vi "ADC Data capture and Process.vi"(0 "ADC Output Read Method":T2(ring)=enum."Read .dat file", 1 "Select the Tab to project":T1(ring)=enum."ADC Sine", 2 "ADC Input":enum16{"Sine Wave", "Ramp / Triangle"}(ring), 3 "No.of samples(SNR)":i32=4096, 4 "Resolution":i32=12, 5 "active edge":i32(ring)=10280, 6 "Inputs for Dyanmic para":T9={"Fundamental Frequency"=100000.0, "Sampling Frequncy"=3999610.0, "No of Harmonics"=9, "Window"=enum."7 Term B-Harris", "Blackman (fundamental power) bins)"=1.0}, 7 "Samples per Channel":i32=4096 caption="No.of Samples(capture)", 8 "Oversampling":bool, 9 "Oversampling ratio":i32, 10 "Drop LSB":bool, 11 "Save data":T15, 12 "Waveform":i64[](array[numeric]), 13 "Path to Read":path=path "C/Users/a0230227/Desktop/save.dat", 14 "Start & Stop Bit":cluster{"Start":i32, "Stop":i32}={"Start"=40, "Stop"=4055}, 15 "length":i32=4096, 24 "path to save":T14={"Path to Save plot"=path "D/Tenor_176P/DYN_PAR_C004/DAT/D001_TEMPP30C_VDD1.2_VDDA3.3_16B_SE_ADCA__vicA_aggX_PLT_CAP_200821_1740_33.jpg", "Path to Raw Data plot"=path "D/Tenor_176P/DYN_PAR_C004/DAT/D001_TEMPP30C_VDD1.2_VDDA3.3_16B_SE_ADCA__vicA_aggX_RAW_DAT_200821_1740_33.csv"}) -> (18 "Min Max":T4, 19 "detected Throughput":dbl, 20 "output cluster":T7, 21 "Dynamic Parameters":T8, 22 "max code":ext, 23 "min code":ext, 25 "Valid Capture":bool)   [LabVIEW 2021] (continued)
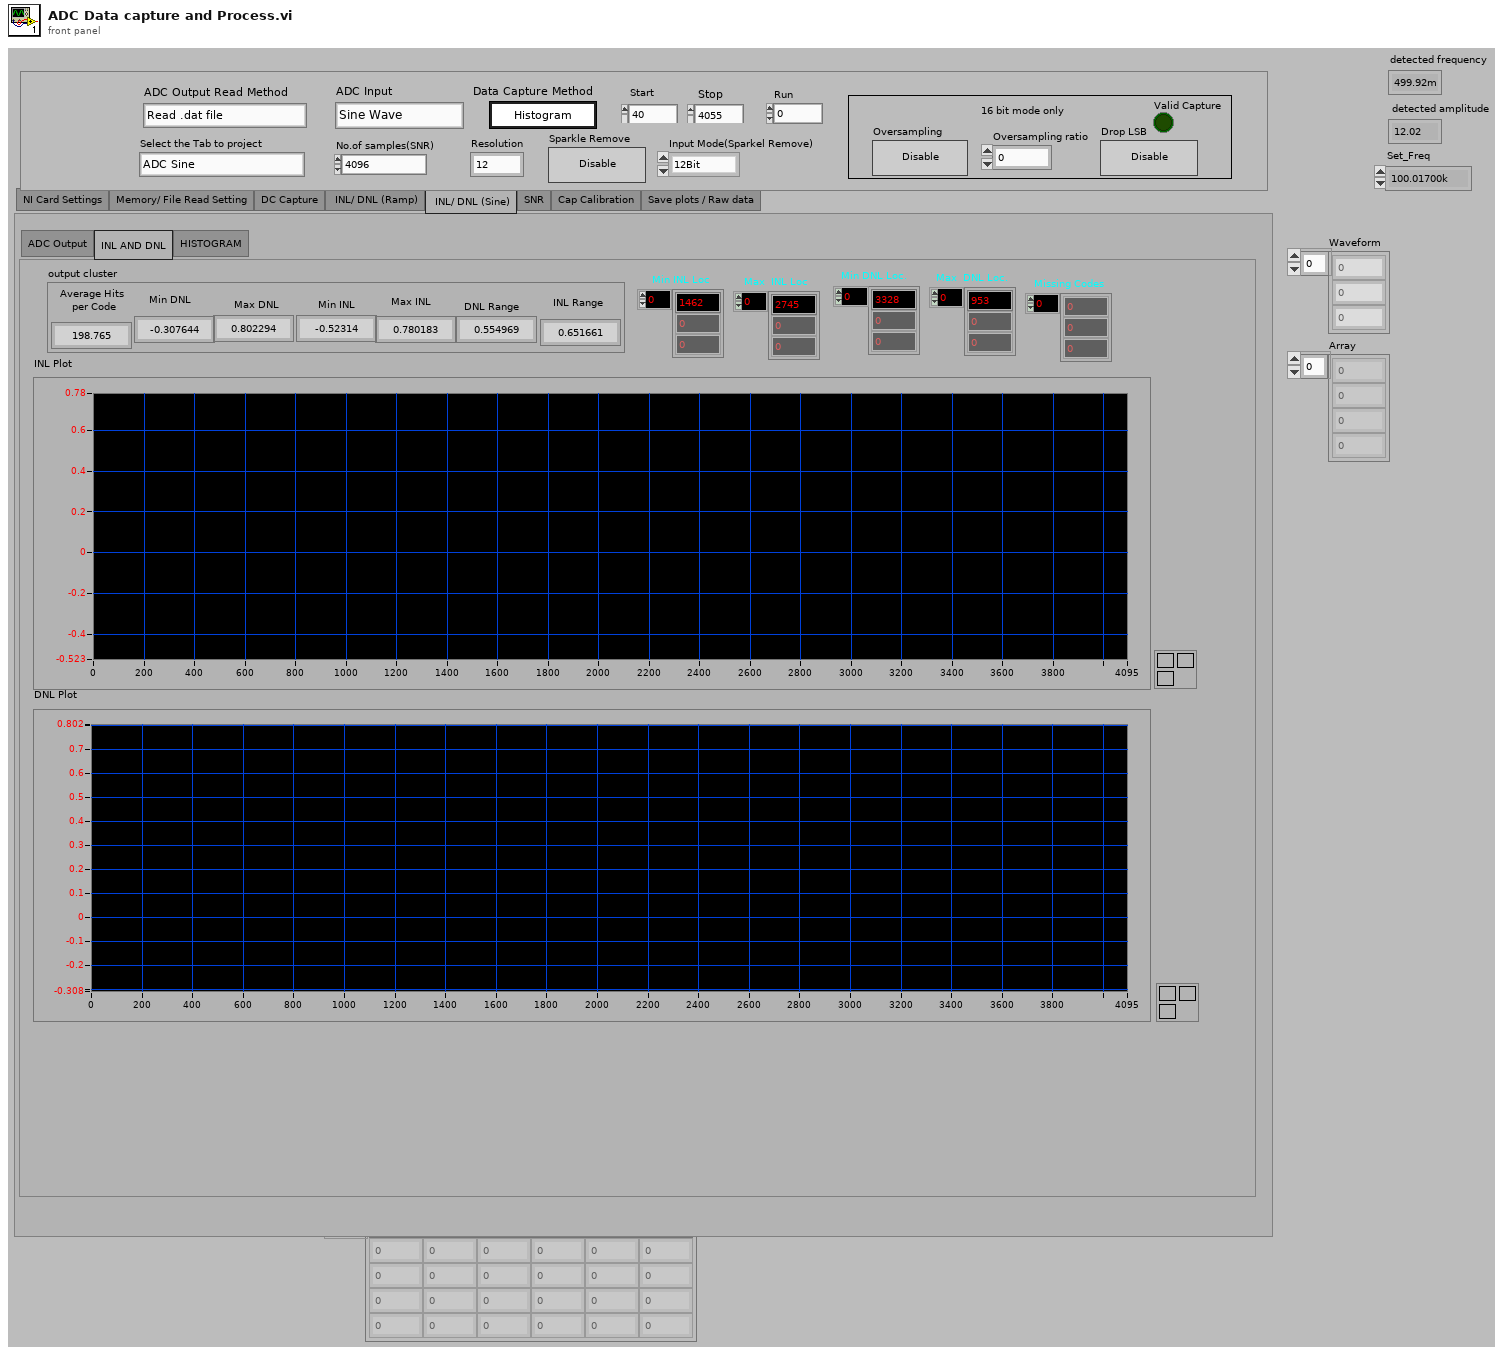
[diagram p1: front panel]
types:
  T1 = enum32{"NI Card Settings", "Memory Read Setting", "DC Capture", "ADC Ramp", "ADC Sine", "SNR", "Cap Calibration"}
  T2 = enum32{"Read from Memory", "Read .dat file", "NI Card Capture", "None"}
  T3 = enum32{"NI Card Settings", "Memory/ File Read Setting", "DC Capture", " INL/ DNL (Ramp)", " INL/ DNL (Sine)", "SNR", "Cap Calibration", "Save plots / Raw data"}
  T4 = cluster{"Min":dbl, "Max":dbl, "delta":dbl, "Average Code":dbl, "Standard Deviation":dbl}
  T5 = cluster{"Min INL":dbl, "Max INL":dbl, "Min DNL":dbl, "Max DNL":dbl, "INL Range":dbl, "DNL Range":dbl, "Avg Hits/Code":dbl}
  T6 = enum32{"ADC Output", "TRIMMED DATA", "INL AND DNL", "HISTOGRAM"}
  T7 = cluster{"Average Hits \nper Code ":dbl, "Min DNL":dbl, "Min INL":dbl, "Max INL":dbl, "Max DNL":dbl, "DNL Range":dbl, "INL Range":dbl}
  T8 = cluster{"SNR":dbl, "SNRD":dbl, "THD":dbl, "ENOB (SNRD)":dbl, "SFDR":dbl, "ENOB (SNR)":dbl, "Noise Power":dbl, "Signal power":dbl}
  T9 = cluster{"Fundamental Frequency":dbl, "Sampling Frequncy":dbl, "No of Harmonics":u8, "Window":enum16{"None ", "Hanning", "Hamming", "Blackman-Harris", "Exact Blackman", "Blackman", "Flat Top", "4 Term B-Harris ", "7 Term B-Harris"}, "Blackman (fundamental power) bins)":dbl}
  T10 = enum32{"ADC Output", "FFT Magnitude plot", " FFT plot"}
  T11 = cluster{"Ideal Power Bin":dbl, "Actual Power Bin":dbl, "Signal Strength (dB)":dbl}
  T12 = cluster{"ADC Reference(V)":dbl, "Bin Width":dbl, "PSRR/ CMRR  ":bool}
  T13 = cluster{"Fundamental Frequnecy (Calculated)":dbl, "Harmonic Frequencies":dbl[], "Harmonic Amplitudes":dbl[]}
  T14 = cluster{"Path to Save plot":path, "Path to Raw Data plot":path}
  T15 = cluster{"Save INL/DNL Plot(Ramp)":bool, "Save SNR Plot":bool, "Save INL/DNL Plot(Sine)":bool, "Save INL/DNL Raw Data(Ramp)":bool, "Save SNR Raw Data":bool, "Save INL/DNL Raw Data(Sine)":bool, "Save DC Raw data":bool, "Save  Raw Data(Sine)":bool}
  T16 = enum16{"Initialize", "Read output", "Post process", "Cap Calib", "Save data", "Exit"}
  T17 = cluster{"Average Hits \nper Code ":dbl, "Min\nDNL":dbl, dbl, dbl, "Max\nDNL":dbl, dbl, dbl}
  T18 = enum16{"None ", "Hanning", "Hamming", "Blackman-Harris", "Exact Blackman", "Blackman", "Flat Top", "4 Term B-Harris ", "7 Term B-Harris"}
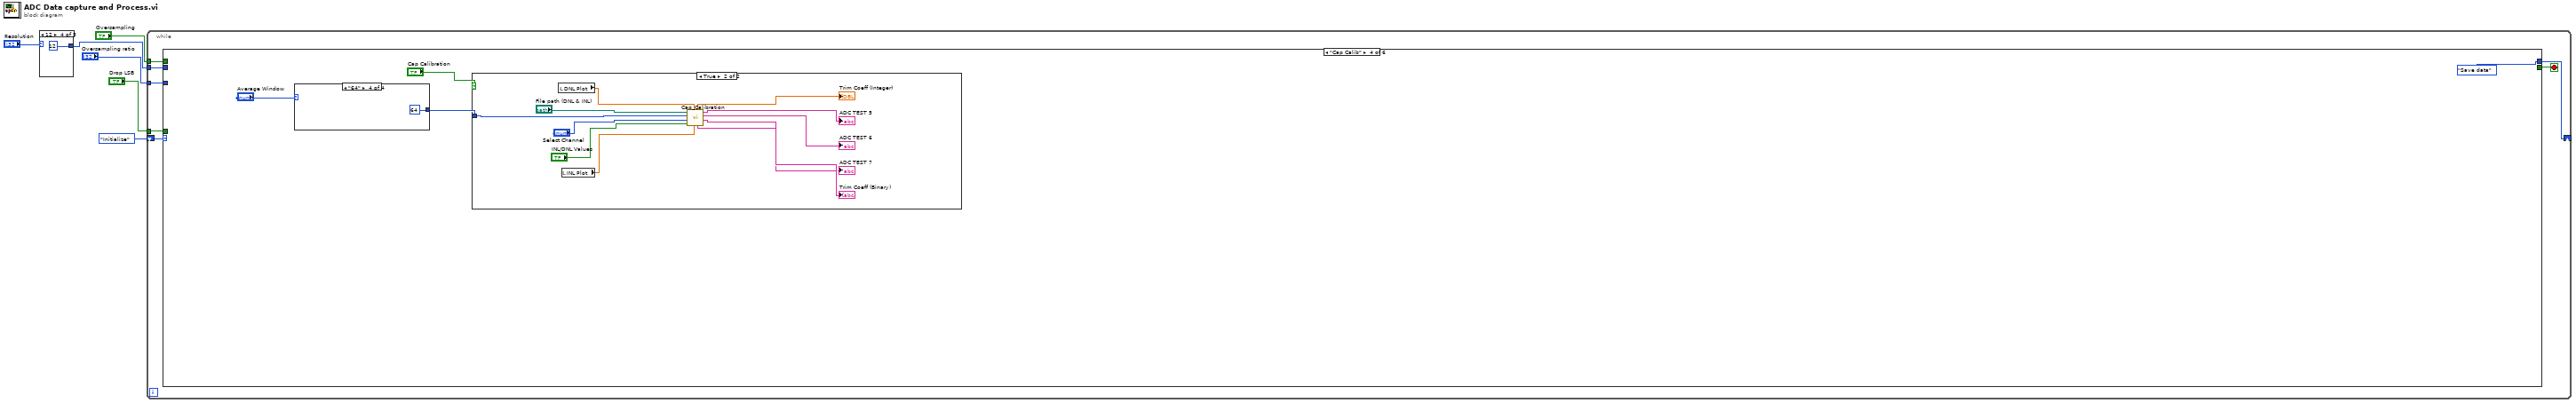
[diagram p0: block diagram]
diagram:
  n1 = case shown="12" "Resolution" {
    tunnel: [18 16 14 12 10] -> w5
    frame 18 {
    }
    frame 16 {
    }
    frame 14, Default {
    }
    frame 12 {
    }
    frame 10 {
    }
  }
  n2 = while {
    shift-right: [w17] -> _
    shift-left: T16."Initialize" -> [w18]
    tunnel: w5 -> [w15]
    tunnel: "Oversampling" -> [w14]
    tunnel: "Drop LSB" -> [w13]
    tunnel: "Oversampling ratio" -> [w12]
    stop <- w16 stop-if-true
    n3 = case shown="\"Cap Calib\"" w18 {
      tunnel: [T16."Read output" w41 w114 T16."Save data" T16."Exit" _] -> w17
      tunnel: [_ _ _ _ _ TRUE] -> w16
      tunnel: w15 -> [_ _ w121 _ _ _]
      tunnel: w14 -> [_ _ w111 _ _ _]
      tunnel: w13 -> [_ _ w113 _ _ _]
      tunnel: w12 -> [_ _ w112 _ _ _]
      frame "Initialize", Default {
        n4 = local read "No.of samples(SNR)"() -> (w19:i32)
        n5 = local write "Samples per Channel"(w19) -> ()
      }
      frame "Read output" {
        w26 = waveform(i64) {"t0"=timestamp(0 s since 1904-01-01), "dt"=1.0, "Y"=[]}  # waveform
        n6 = case shown="\"NI Card Capture\", Default" "ADC Output Read Method" {
          tunnel: [w51 _ w70 "Waveform"] -> w27
          tunnel: [T16."Post process" _ T16."Post process" T16."Post process"] -> w41
          frame "Read .dat file" {
            w50 = 0  # index
            w56 = 8192 ("index")
            w61 = 1 ("index")
            n7 = call-poly <vilib>:"Read From Spreadsheet File.vi"("delimiter (\\t)"="Delimiter (\\t)", "file path (dialog if empty)"="Path to Read") -> ("all rows"=w63:i64[][])  [unwired: 5 in, 4 out]
            n8 = Index Array(array=w63, index (col)=0 ("disabled index (col)")) -> (element=w54:i64[])  [unwired: 1 in]
            n9 = Split 1D Array(array=w54, index=w61) -> (second subarray=w52:i64[])  [unwired: 1 out]
            n10 = Multiply(x=w56, y=1) -> (x*y=w59:i32)
            n11 = Multiply(x=2 ("y"), y=w56) -> (x*y=w57:i32)
            n12 = Multiply(x=w56, y=3) -> ()  [unwired: 1 out]
            n13 = Array Subset(array=w52, index=w61, length=w56) -> ()  [unwired: 1 out]
            n14 = Array Subset(array=w52, index=w59, length=w56) -> ()  [unwired: 1 out]
            n15 = Array Subset(array=w52, index=w57, length=w56) -> ()  [unwired: 1 out]
            n16 = Array Subset(array=w52, index=w50, length="length") -> (w51:i64[])
          }
          frame "None" {
          }
          frame "NI Card Capture", Default {
            n17 = case shown="\"Sine Wave\", Default" "ADC Input" {
              tunnel: "Port" -> [w87 w97]
              tunnel: "Source" -> [w86 w96]
              tunnel: "Rate" -> [w85 w95]
              tunnel: "Timeout" -> [w84 w94]
              tunnel: [_ w92] -> w69
              tunnel: [w80 w93] -> w70
              tunnel: "No.of samples(SNR)" -> [w83 w91]
              tunnel: "Samples per Channel" -> [w81 w90]
              tunnel: "Sparkle Remove" -> [w79 _]
              tunnel: "active edge" -> [w78 w88]
              frame "Sine Wave", Default {
                n18 = call "DATA_CAPTURE_SNR.vi"("Port"=w87, "Source"=w86, "No. of samples to process"=w83, "Samples per Channel"=w81, "Rate"=w85, "active edge"=w78, "timeout"=w84, "Histogram Capture Method SNR"=w79, "NI card Cont/Single Capture"=FALSE ("Histogram Capture Method SNR")) -> ("Waveform"=w80:u32[])  [unwired: 5 in, 5 out]
              }
              frame "Ramp / Triangle" {
                n19 = disable-structure shown="Disabled" {
                  disable-tunnel: w97 -> [w108 _]
                  disable-tunnel: w96 -> [w107 _]
                  disable-tunnel: w95 -> [w106 _]
                  disable-tunnel: w94 -> [w105 _]
                  disable-tunnel: [w104 _] -> w93
                  disable-tunnel: [w103 _] -> w92
                  disable-tunnel: w91 -> [w102 _]
                  disable-tunnel: w90 -> [w100 _]
                  disable-tunnel: FALSE ("Histogram Capture Method SNR") -> [w99 _]
                  disable-tunnel: w88 -> [w98 _]
                  frame Disabled {
                    n20 = call "DATA_CAPTURE_SNR.vi"("Port"=w108, "Source"=w107, "No. of samples to process"=w102, "Samples per Channel"=w100, "Rate"=w106, "active edge"=w98, "timeout"=w105, "Histogram Capture Method SNR"=w99, "NI card Cont/Single Capture"=FALSE ("Histogram Capture Method SNR")) -> ("Waveform"=w104:u32[], "Trimmed Wave"=w103:u32[])  [unwired: 5 in, 4 out]
                  }
                  frame Enabled {
                  }
                }
              }
            }
            "Trimmed Wave" <- w69
          }
          frame "Read from Memory" {
          }
        }
        "Ramp Waveform" <- w27
        "Sine Waveform" <- w27
        "Read Data from Device" <- w27
        "Captured Data" <- w27
        "DC capture" <- w27
        n21 = Bundle By Name(cluster=w26, "Y"=w27) -> (w25:waveform(i64))
        n22 = Array Size(array=w27) -> (size(s)=w37:i32)
        n23 = Array Max & Min(array=w27) -> (max value=→"max code":i64, min value=→"min code":i64)  [unwired: 2 out]
        n24 = Decrement(x=w37) -> (x-1=w36:i32)
        n25 = call-poly <vilib>:"Extract Single Tone Information.vi"("time signal in"=w25) -> ("detected amplitude"=→"detected amplitude":dbl, "detected frequency"=w22:dbl)  [unwired: 5 in, 4 out]
        "detected frequency" <- w22
        n26 = for {
          N: w36 -> [_]
          tunnel: w27 -> [w48]
          tunnel: [w42] -> w34 mode=indexing
          i -> [w46]
          n27 = Increment(x=w46) -> (x+1=w47:i32)
          n28 = Index Array(array=w48, index=w46) -> (element=w44:i64)
          n29 = Index Array(array=w48, index=w47) -> (element=w45:i64)
          n30 = Subtract(x=w45, y=w44) -> (x-y=w43:i64)
          n31 = Absolute Value(x=w43) -> (abs(x)=w42:i64)
        }
        n32 = Divide(x="Set_Freq", y=w22) -> (x/y=→"detected Throughput":dbl)
        n33 = Add Array Elements(numeric array=w34) -> (sum=w32:i64)
        n34 = Array Max & Min(array=w34) -> (max value=w29:i64)  [unwired: 3 out]
        n35 = Array Size(array=w34) -> (size(s)=w31:i32)
        n36 = Divide(x=w32, y=w31) -> (x/y=w33:dbl)
        n37 = Multiply(x=2.0, y=w33) -> (x*y=w28:dbl)
        n38 = Less?(x=w29, y=w28) -> (x < y?=→"Valid Capture":bool)
      }
      frame "Post process" {
        n39 = local read "Select the Tab to project"() -> (w127:T1)
        n40 = local read "Read Data from Device"() -> (w118:dbl[])
        n41 = local read "No.of samples(SNR)"() -> (w120:i32)
        n42 = Equal?(x=w127, y=T1."Cap Calibration" ("Select the Tab to project")) -> (x = y?=w128:bool)
        n43 = Unbundle By Name("Start & Stop Bit") -> ("Start"=w123:i32, "Stop"=w122:i32)
        n44 = Select(t=T1."ADC Sine" ("Select the Tab to project"), s=w128, f=w127) -> (s? t:f=w126:T1)
        n45 = case shown="\"SNR\"" w126 {
          tunnel: w118 -> [w133 w249 w321 w386]
          tunnel: "Data Capture Method" -> [w130 w247 w354 _]
          tunnel: w123 -> [_ w246 w353 _]
          tunnel: w122 -> [_ w245 w352 _]
          tunnel: w121 -> [_ w248 w351 w385]
          tunnel: w120 -> [_ _ _ w387]
          tunnel: [_ w244 w339 _] -> w119
          tunnel: [T16."Save data" T16."Save data" T16."Cap Calib" T16."Save data"] -> w114
          tunnel: w111 -> [_ _ w318 w383]
          tunnel: w113 -> [_ _ w317 w382]
          tunnel: w112 -> [_ _ w319 w381]
          frame "DC Capture", Default {
            n46 = property on="Raw Data CH2" class="Arr (strict)"("Visible"="CH Swtich (To see other CH O/P)") -> ()  [unwired: 2 in, 2 out]
            n47 = property on="Standard Deviation (CH2)" class="DigNum (strict)"("Visible"="CH Swtich (To see other CH O/P)") -> ()  [unwired: 2 in, 2 out]
            n48 = property on="Raw Data CH1" class="Arr (strict)"("Visible"="CH Swtich (To see other CH O/P)") -> ()  [unwired: 2 in, 2 out]
            n49 = property on="Average Code (CH2)" class="DigNum (strict)"("Visible"="CH Swtich (To see other CH O/P)") -> ()  [unwired: 2 in, 2 out]
            n50 = case shown="False" w130 {
              tunnel: w133 -> [w136 w204]
              tunnel: "CH Swtich (To see other CH O/P)" -> [w135 _]
              tunnel: [w134 w190] -> w129
              frame False {
                n51 = case shown="True" w135 {
                  tunnel: w136 -> [w141 w178]
                  tunnel: [w137 w170] -> w134
                  frame True {
                    w147 = 10 ("index")
                    w160 = 10 ("index")
                    n52 = Decimate 1D Array(w141) -> (w157:dbl[], w148:dbl[])
                    "Raw Data CH2" <- w157
                    "Raw Data CH1" <- w148
                    n53 = Split 1D Array(array=w157, index=w160) -> (second subarray=w159:dbl[])  [unwired: 1 out]
                    n54 = Split 1D Array(array=w148, index=w147) -> (second subarray=w156:dbl[])  [unwired: 1 out]
                    n55 = Array Size(array=w159) -> (size(s)=w161:i32)
                    n56 = Array Size(array=w156) -> (size(s)=w155:i32)
                    n57 = Subtract(x=w161, y=w160) -> (x-y=w164:i32)
                    n58 = Subtract(x=w155, y=w147) -> (x-y=w145:i32)
                    n59 = Split 1D Array(array=w159, index=w164) -> (first subarray=w163:dbl[])  [unwired: 1 out]
                    n60 = Split 1D Array(array=w156, index=w145) -> (first subarray=w153:dbl[])  [unwired: 1 out]
                    n61 = Array Size(array=w163) -> (size(s)=w162:i32)
                    n62 = Array Size(array=w153) -> (size(s)=w154:i32)
                    n63 = To Double Precision Float(number=w163) -> (double precision float=w165:dbl[])
                    n64 = To Double Precision Float(number=w153) -> (double precision float=w144:dbl[])
                    n65 = Add Array Elements(numeric array=w165) -> (sum=w169:dbl)
                    n66 = Add Array Elements(numeric array=w144) -> (sum=w149:dbl)
                    n67 = Divide(x=w169, y=w162) -> (x/y=w142:dbl)
                    "Average Code (CH2)" <- w142
                    n68 = Divide(x=w149, y=w154) -> (x/y=w139:dbl)
                    n69 = Subtract(x=w165, y=w142) -> (x-y=w168:dbl[])
                    n70 = Subtract(x=w144, y=w139) -> (x-y=w150:dbl[])
                    n71 = Square(x=w168) -> (x^2=w167:dbl[])
                    n72 = Square(x=w150) -> (x^2=w151:dbl[])
                    n73 = Add Array Elements(numeric array=w167) -> (sum=w166:dbl)
                    n74 = Add Array Elements(numeric array=w151) -> (sum=w152:dbl)
                    n75 = Divide(x=w166, y=w162) -> (x/y=w158:dbl)
                    n76 = Divide(x=w152, y=w154) -> (x/y=w146:dbl)
                    n77 = Square Root(x=w158) -> (sqrt(x)=→"Standard Deviation (CH2)":dbl)
                    n78 = Square Root(x=w146) -> (sqrt(x)=w138:dbl)
                    n79 = local read "Min Max"() -> (w140:T4)
                    n80 = Bundle By Name(cluster=w140, "Average Code"=w139, "Standard Deviation"=w138) -> (w137:T4)
                  }
                  frame False {
                    w182 = 10 ("index")
                    n81 = Split 1D Array(array=w178, index=w182) -> (second subarray=w189:dbl[])  [unwired: 1 out]
                    n82 = Array Size(array=w189) -> (size(s)=w188:i32)
                    n83 = Subtract(x=w188, y=w182) -> (x-y=w180:i32)
                    n84 = Split 1D Array(array=w189, index=w180) -> (first subarray=w177:dbl[])  [unwired: 1 out]
                    n85 = Array Size(array=w177) -> (size(s)=w187:i32)
                    n86 = To Double Precision Float(number=w177) -> (double precision float=w179:dbl[])
                    n87 = Add Array Elements(numeric array=w179) -> (sum=w183:dbl)
                    n88 = Divide(x=w183, y=w187) -> (x/y=w172:dbl)
                    n89 = Subtract(x=w179, y=w172) -> (x-y=w184:dbl[])
                    n90 = Square(x=w184) -> (x^2=w185:dbl[])
                    n91 = Add Array Elements(numeric array=w185) -> (sum=w186:dbl)
                    n92 = Divide(x=w186, y=w187) -> (x/y=w181:dbl)
                    n93 = Array Max & Min(array=w177) -> (max value=w174:dbl, min value=w173:dbl)  [unwired: 2 out]
                    n94 = local read "Min Max"() -> (w176:T4)
                    n95 = Subtract(x=w174, y=w173) -> (x-y=w175:dbl)
                    n96 = Square Root(x=w181) -> (sqrt(x)=w171:dbl)
                    n97 = Bundle By Name(cluster=w176, "Standard Deviation"=w171, "Average Code"=w172, "Max"=w174, "Min"=w173, "delta"=w175) -> (w170:T4)
                  }
                }
              }
              frame True {
                n98 = for {
                  tunnel: w204 -> [w237] mode=indexing
                  shift-right: [w241] -> w213
                  shift-left: 0.0 ("x*y") -> [w242]
                  tunnel: w204 -> [w240]
                  tunnel: [w239] -> w212
                  shift-right: [w228] -> _
                  shift-left: TRUE ("x != 0?") -> [w235]
                  shift-right: [w231] -> w195
                  shift-left: i32[] [] -> [w232]
                  i -> [w234]
                  n99 = Add Array Elements(numeric array=w240) -> (sum=w239:dbl)
                  n100 = Not Equal To 0?(x=w237) -> (x != 0?=w236:bool)
                  n101 = Multiply(x=w237, y=w234) -> (x*y=w238:dbl)
                  n102 = Build Array (concatenate)(w232, w234) -> (w233:i32[])
                  n103 = And(x=w235, y=w236) -> (x .and. y?=w230:bool)
                  n104 = Add(x=w242, y=w238) -> (x+y=w241:dbl)
                  n105 = Select(t=w233, s=w230, f=w232) -> (s? t:f=w231:i32[])
                  n106 = Select(t=FALSE ("x != 0?"), s=w230, f=TRUE ("x != 0?")) -> (s? t:f=w228:bool)
                }
                n107 = Divide(x=w213, y=w212) -> (x/y=w191:dbl)
                n108 = Array Size(array=w195) -> (size(s)=w193:i32)
                n109 = Index Array(array=w195, index=0) -> (element=w196:i32)
                n110 = Split 1D Array(array=w204, index=w196) -> (second subarray=w199:dbl[])  [unwired: 1 out]
                n111 = Subtract(x=w193, y=15 ("x")) -> (x-y=w192:i32)
                n112 = Array Max & Min(array=w199) -> (max index (indices)=w207:i32)  [unwired: 3 out]
                n113 = Greater?(x=w207, y=w192) -> (0:w208:bool)
                n114 = case shown="True" w208 {
                  tunnel: w207 -> [w216 w223]
                  tunnel: [w215 w223] -> w203
                  tunnel: 10 ("y") -> [w220 w222]
                  tunnel: w199 -> [w219 w226]
                  tunnel: [w216 w225] -> w202
                  tunnel: [_ w221] -> w197
                  frame True {
                    n115 = Subtract(x=w216, y=w220) -> (x-y=w217:i32)
                    n116 = Split 1D Array(array=w219, index=w217) -> (first subarray=w218:dbl[])  [unwired: 1 out]
                    n117 = Array Max & Min(array=w218) -> (max index (indices)=w215:i32)  [unwired: 3 out]
                  }
                  frame False {
                    n118 = Add(x=w223, y=w222) -> (x+y=w221:i32)
                    n119 = Split 1D Array(array=w226, index=w221) -> (second subarray=w224:dbl[])  [unwired: 1 out]
                    n120 = Array Max & Min(array=w224) -> (max index (indices)=w225:i32)  [unwired: 3 out]
                  }
                }
                n121 = Add(x=w196, y=w203) -> (x+y=w200:i32)
                n122 = Compound Arithmetic op=ADD(w196, w202, w197) -> (w201:i32)
                n123 = Subtract(x=w201, y=w200) -> (x-y=w206:i32)
                n124 = local read "Min Max"() -> (w211:T4)
                n125 = Bundle By Name(cluster=w211, "Average Code"=w191, "Min"=w200, "Max"=w201, "delta"=w206) -> (w190:T4)
              }
            }
            "Min Max" <- w129
          }
          frame "ADC Ramp" {
            n126 = stacked-sequence {
              seq-local: [w251 _ _] -> [_ w275 _]
              seq-local: [_ w271 _] -> [_ _ w301]
              seq-local: [_ w270 _] -> [_ _ w300]
              seq-local: [_ w269 _] -> [_ _ w289]
              seq-local: [w252 _ _] -> [_ w268 _]
              tunnel: w249 -> [w254 _ _]
              tunnel: w248 -> [w256 _ _]
              tunnel: w247 -> [w255 _ _]
              tunnel: w246 -> [_ w274 _]
              tunnel: w245 -> [_ w273 _]
              tunnel: [w251 _ _] -> w244
              frame #0 {
                n127 = local read "Trimmed Wave"() -> (w250:u32[])
                n128 = Scale By Power Of 2(n=w256, x=ext 1.0) -> (x*2^n=w252:ext)
                n129 = Initialize Array(0 ("element"), w252) -> (w260:i32[])
                n130 = for {
                  shift-right: [w263] -> w253
                  shift-left: w260 -> [w264]
                  tunnel: 0.0 -> [w262]
                  tunnel: w250 -> [w261] mode=indexing
                  n131 = Subtract(x=w261, y=w262) -> (x-y=w265:dbl)
                  n132 = in-place {
                    n133 = in-place-array #1(w264, w265) -> (w267:i32)
                    n134 = Increment(x=w267) -> (x+1=w266:i32)
                    n135 = in-place-array #1(w266) -> (w263:i32[])  [unwired: 1 out]
                  }
                }
                n136 = Select(t=w254, s=w255, f=w253) -> (s? t:f=w251:dbl[])
                "Histogram waveform" <- w251
              }
              frame #1 {
                n137 = Subtract(x=w273, y=w274) -> (x-y=w276:i32)
                n138 = Split 1D Array(array=w275, index=w274) -> (second subarray=w283:dbl[])  [unwired: 1 out]
                n139 = Split 1D Array(array=w283, index=w276) -> (first subarray=w277:dbl[])  [unwired: 1 out]
                n140 = Add Array Elements(numeric array=w277) -> (sum=w280:dbl)
                n141 = Array Size(array=w277) -> (size(s)=w279:i32)
                n142 = Divide(x=w280, y=w279) -> (x/y=w269:dbl)
                n143 = Initialize Array(w269, w268) -> (w278:dbl[])
                n144 = Replace Array Subset(array=w278, new element=w277, index=w274) -> (w282:dbl[])
                n145 = Divide(x=w282, y=w269) -> (x/y=w281:dbl[])
                n146 = Decrement(x=w281) -> (x-1=w271:dbl[])
                "DNL_Ramp" <- w271
                n147 = for {
                  shift-right: [w285] -> _
                  shift-left: 0.0 ("x") -> [w286]
                  tunnel: [w285] -> w270 mode=indexing
                  tunnel: w271 -> [w284] mode=indexing
                  n148 = Add(x=w286, y=w284) -> (x+y=w285:dbl)
                }
                "INL_Ramp" <- w270
              }
              frame #2 {
                n149 = Array Max & Min(array=w301) -> (max value=w292:dbl, min value=w293:dbl)  [unwired: 2 out]
                n150 = Array Max & Min(array=w300) -> (max value=w294:dbl, min value=w295:dbl)  [unwired: 2 out]
                n151 = Subtract(x=w292, y=w293) -> (x-y=w297:dbl)
                n152 = Subtract(x=w294, y=w295) -> (x-y=w298:dbl)
                n153 = local read "Static Parameters (Ramp)"() -> (w288:T5)
                n154 = Divide(x=w297, y=2.0) -> (x/y=w290:dbl)
                n155 = Divide(x=w298, y=2.0) -> (x/y=w291:dbl)
                n156 = disable-structure shown="Enabled" {
                  disable-tunnel: w295 -> [w316 _]
                  disable-tunnel: w294 -> [w315 _]
                  disable-tunnel: w293 -> [w314 _]
                  disable-tunnel: w292 -> [w313 _]
                  disable-tunnel: w291 -> [w304 _]
                  disable-tunnel: w290 -> [w303 _]
                  disable-tunnel: w289 -> [w302 _]
                  frame Disabled {
                    n157 = Increment(x="Run") -> (x+1=w305:dbl)
                    n158 = local write "Run"(w305) -> ()
                    n159 = Build Array(w305, w316, w315, w314, w313, w304, w303, w302) -> (w312:dbl[])
                    n160 = call-poly <vilib>:"Write To Spreadsheet File.vi"("delimiter (\\t)"="," ("delimiter (\\t)"), "transpose? (no:F)"=FALSE, "format (%.3f)"="%.4f", "append to file? (new file:F)"=TRUE, "1D data"=w312, "file path (dialog if empty)"=path "D:/FALCON/ADC/Raw_Data/runtorun.csv") -> ()  [unwired: 2 in, 1 out]
                  }
                  frame Enabled {
                  }
                }
                n161 = Bundle By Name(cluster=w288, "Max INL"=w294, "Min INL"=w295, "Max DNL"=w292, "Min DNL"=w293, "INL Range"=w291, "DNL Range"=w290, "Avg Hits/Code"=w289) -> (→"Static Parameters (Ramp)":T5)
              }
            }
          }
          frame "ADC Sine" {
            n162 = case shown="True" w318 {
              tunnel: w321 -> [w356 w364]
              tunnel: [w357 w362] -> w320
              tunnel: w319 -> [_ w363]
              tunnel: w317 -> [w355 _]
              frame False {
                n163 = case shown="True" w355 {
                  tunnel: w356 -> [w358 w360]
                  tunnel: [w358 w359] -> w357
                  frame False {
                  }
                  frame True {
                    n164 = Divide(x=w360, y=2.0) -> (x/y=w359:dbl[])
                  }
                }
              }
              frame True {
                n165 = Array Size(array=w364) -> (size(s)=w366:i32)
                n166 = Divide(x=w366, y=w363) -> (x/y=w365:dbl)
                n167 = for {
                  N: w365 -> [_]
                  tunnel: w364 -> [w373]
                  tunnel: w363 -> [w368]
                  tunnel: [w367] -> w362 mode=indexing
                  i -> [w372]
                  n168 = Multiply(x=w368, y=w372) -> (x*y=w371:i32)
                  n169 = Array Subset(array=w373, index=w371, length=w368) -> (w370:dbl[])
                  n170 = Add Array Elements(numeric array=w370) -> (sum=w369:dbl)
                  n171 = Divide(x=w369, y=w368) -> (x/y=w367:dbl)
                }
              }
            }
            n172 = call "Sinewave_Linearity_trial_F027.vi"("Array"=w320, "Histogram Capture Method"=w354, "L code"=w353, "UCode"=w352, "Resolution"=w351, "Histogram: h(x)"=w320) -> ("Average Hits \nper Code"=w329:dbl, "Max\nDNL"=w325:dbl, "Min\nDNL"=w328:dbl, "Missing Codes"=→"Missing Codes":i32[], "Max  DNL Loc."=→"Max  DNL Loc.":i32[], "Min DNL Loc."=→"Min DNL Loc.":i32[], "Max  INL Loc"=→"Max  INL Loc":i32[], "Min INL Loc"=→"Min INL Loc":i32[], "Histogram Plot"=w341:dbl[][], "DNL Plot"=w337:dbl[], "INL Plot"=w330:dbl[])  [unwired: 1 in, 2 out]
            "Histogram Plot" <- w341
            "DNL Plot" <- w337
            "INL Plot" <- w330
            n173 = for {
              tunnel: w337 -> [w380] mode=indexing
              tunnel: [w376] -> w336 mode=indexing
              shift-right: [w375] -> _
              shift-left: 16384 ("f") -> [w374]
              i -> [w377]
              n174 = Increment(x=w374) -> (x+1=w375:i32)
              n175 = Greater?(x=w380, y=0.9) -> (0:w378:bool)
              n176 = Select(t=w377, s=w378, f=w374) -> (s? t:f=w376:i32)
            }
            n177 = Subtract(x=w325, y=w328) -> (x-y=w348:dbl)
            n178 = Array Max & Min(array=w330) -> (max value=w326:dbl, min value=w327:dbl)  [unwired: 2 out]
            n179 = Index Array(array=w341, index (col)=1 ("disabled index (col)")) -> (element=w339:dbl[])  [unwired: 1 in]
            n180 = Subtract(x=w326, y=w327) -> (x-y=w350:dbl)
            n181 = Divide(x=w348, y=2.0) -> (x/y=w324:dbl)
            n182 = Divide(x=w350, y=2.0) -> (x/y=w323:dbl)
            n183 = Bundle("Average Hits \nper Code"=w329, "Min\nDNL"=w328, w327, w326, "Max\nDNL"=w325, w324, w323) -> (→"output cluster":T17)  [unwired: 1 in]
            n184 = Sort 1D Array(array=w336) -> (sorted array=w332:i32[])
            n185 = Search 1D Array(1D array=w332, element=16384) -> (index of element=w333:i32)  [unwired: 1 in]
            n186 = Array Subset(array=w332, length=w333) -> (→"Array":i32[])  [unwired: 1 in]
          }
          frame "SNR" {
            n187 = stacked-sequence {
              seq-local: [w408 _ _] -> [_ w469 _]
              seq-local: [w407 _ _] -> [_ _ w494]
              seq-local: [w401 _ _] -> [_ _ w497]
              seq-local: [w400 _ _] -> [_ _ w493]
              seq-local: [w399 _ _] -> [_ _ w492]
              tunnel: w387 -> [w420 _ w495]
              tunnel: w386 -> [w402 _ _]
              tunnel: w385 -> [w404 _ _]
              tunnel: w383 -> [w391 _ _]
              tunnel: w382 -> [w390 _ _]
              tunnel: w381 -> [w389 _ _]
              frame #0 {
                n188 = Unbundle By Name("PSRR/CMRR Input") -> ("ADC Reference(V)"=w403:dbl, "PSRR/ CMRR"=w399:bool)
                n189 = case shown="True" w399 {
                  tunnel: 1.0 ("x") -> [_ w455]
                  tunnel: w404 -> [_ w454]
                  tunnel: w403 -> [_ w452]
                  tunnel: w402 -> [w448 w450]
                  tunnel: [w448 w449] -> w393
                  frame False {
                  }
                  frame True {
                    n190 = Scale By Power Of 2(n=w454, x=w455) -> (x*2^n=w453:dbl)
                    n191 = Divide(x=w452, y=w453) -> (x/y=w451:dbl)
                    n192 = Multiply(x=w450, y=w451) -> (x*y=w449:dbl[])
                  }
                }
                n193 = case shown="True" w391 {
                  tunnel: w393 -> [w430 w438]
                  tunnel: [w431 w436] -> w392
                  tunnel: w389 -> [_ w437]
                  tunnel: w390 -> [w429 _]
                  frame False {
                    n194 = case shown="True" w429 {
                      tunnel: w430 -> [w432 w434]
                      tunnel: [w432 w433] -> w431
                      frame False {
                      }
                      frame True {
                        n195 = Divide(x=w434, y=2.0) -> (x/y=w433:dbl[])
                      }
                    }
                  }
                  frame True {
                    n196 = Array Size(array=w438) -> (size(s)=w440:i32)
                    n197 = Divide(x=w440, y=w437) -> (x/y=w439:dbl)
                    n198 = for {
                      N: w439 -> [_]
                      tunnel: w438 -> [w447]
                      tunnel: w437 -> [w442]
                      tunnel: [w441] -> w436 mode=indexing
                      i -> [w446]
                      n199 = Multiply(x=w442, y=w446) -> (x*y=w445:i32)
                      n200 = Array Subset(array=w447, index=w445, length=w442) -> (w444:dbl[])
                      n201 = Add Array Elements(numeric array=w444) -> (sum=w443:dbl)
                      n202 = Divide(x=w443, y=w442) -> (x/y=w441:dbl)
                    }
                  }
                }
                n203 = Unbundle By Name("Inputs for Dyanmic para") -> ("Window"=w418:T18, "Sampling Frequncy"=w407:dbl, "Fundamental Frequency"=w401:dbl, "No of Harmonics"=w408:u8, "Blackman (fundamental power) bins)"=w417:dbl)
                n204 = Reciprocal(x=w407) -> (1/x=w422:dbl)
                n205 = call-poly <vilib>:"Scaled Time Domain Window.vi"("window"=w418, "X"=w392) -> ("Windowed X"=w426:dbl[])  [unwired: 7 in, 2 out]
                n206 = local read "Dynamic Parameters"() -> (w416:T8)
                n207 = call <vilib>:"Auto Power Spectrum.vi"("dt"=w422, "Signal (V)"=w426) -> ("Power Spectrum (V^2 rms)"=w421:dbl[])  [unwired: 1 out]
                n208 = Logarithm Base 10(1:w421) -> (0:w428:dbl[])
                n209 = call "Calculate_SNR_THD.vi"("Auto Power Spectrum"=w421, "frame size"=w420, "# harmonics"=w408, "window"=w418, "sampling rate"=w407, "fundamental frequency"=w401, "Blackman\n (fundamental power bins)"=w417) -> ("% THD"=w415:dbl, "ENOB(SNRD)"=w410:dbl, "% THD + Noise"=w388:dbl, "ENOB(SNR)"=w411:dbl, "Noise Power"=w414:dbl, "Fundamental frequency Calculated"=w396:dbl, "SNR"=w413:dbl, "Signal power"=w412:dbl, "Harmonic Amplitudes"=w423:dbl[], "Harmonic Frequencies"=w398:dbl[])  [unwired: 3 in]
                n210 = Bundle By Name(cluster=w416, "THD"=w415, "SNRD"=w388, "Noise Power"=w414, "SNR"=w413, "Signal power"=w412, "ENOB (SNR)"=w411, "ENOB (SNRD)"=w410) -> (→"Dynamic Parameters":T8)
                n211 = Logarithm Base 10(1:w423) -> (0:w425:dbl[])
                n212 = Multiply(x=10.0, y=w428) -> (x*y=w400:dbl[])
                "FFT Magnitude Plot (dB)" <- w400
                n213 = local read "Harmonic Details"() -> (w394:T13)
                n214 = Multiply(x=20, y=w425) -> (x*y=w397:dbl[])
                n215 = Bundle By Name(cluster=w394, "Fundamental Frequnecy (Calculated)"=w396, "Harmonic Frequencies"=w398, "Harmonic Amplitudes"=w397) -> (→"Harmonic Details":T13)
              }
              frame #1 {
                n216 = local read "Harmonic Details"() -> (w457:T13)
                n217 = Unbundle By Name(w457) -> ("Harmonic Amplitudes"=w456:dbl[])
                n218 = Decrement(x=w469) -> (x-1=w475:u8)
                n219 = Index Array(array=w456, index=0) -> (element=w471:dbl)
                n220 = Array Subset(array=w456, index=1, length=w475) -> (w473:dbl[])
                n221 = Array Max & Min(array=w473) -> (max value=w470:dbl)  [unwired: 3 out]
                n222 = local read "Dynamic Parameters"() -> (w468:T8)
                n223 = Subtract(x=w471, y=w470) -> (x-y=w467:dbl)
                n224 = Bundle By Name(cluster=w468, "SFDR"=w467) -> (w466:T8)
                n225 = local write "Dynamic Parameters"(w466) -> ()
                n226 = Unbundle By Name(w466) -> ("SNR"=w465:dbl, "SNRD"=w464:dbl, "THD"=w463:dbl, "SFDR"=w462:dbl, "ENOB (SNR)"=w461:dbl, "ENOB (SNRD)"=w460:dbl, "Noise Power"=w459:dbl, "Signal power"=w458:dbl)
                n227 = disable-structure shown="Enabled" {
                  disable-tunnel: w465 -> [w491 _]
                  disable-tunnel: w464 -> [w490 _]
                  disable-tunnel: w460 -> [w478 _]
                  disable-tunnel: w463 -> [w481 _]
                  disable-tunnel: w462 -> [w480 _]
                  disable-tunnel: w461 -> [w479 _]
                  disable-tunnel: w459 -> [w477 _]
                  disable-tunnel: w458 -> [w476 _]
                  frame Disabled {
                    n228 = local read "Run"() -> (w482:dbl)
                    n229 = Increment(x=w482) -> (x+1=w483:dbl)
                    n230 = local write "Run"(w483) -> ()
                    n231 = Build Array(w483, w491, w490, w481, w480, w479, w478, w477, w476) -> (w489:dbl[])
                    n232 = call-poly <vilib>:"Write To Spreadsheet File.vi"("delimiter (\\t)"="," ("delimiter (\\t)"), "transpose? (no:F)"=FALSE, "format (%.3f)"="%.4f", "append to file? (new file:F)"=TRUE, "1D data"=w489, "file path (dialog if empty)"=path "D:/FALCON/ADC/Raw_Data/runtorun.csv") -> ()  [unwired: 2 in, 1 out]
                  }
                  frame Enabled {
                  }
                }
              }
              frame #2 {
                n233 = local read "FFT Magnitude Plot (dB)"() -> (w504:dbl[])
                n234 = Array Size(array=w504) -> (size(s)=w503:i32)
                n235 = Divide(x=w494, y=2.0) -> (x/y=w501:dbl)
                n236 = for {
                  N: w503 -> [_]
                  tunnel: w504 -> [w547]
                  tunnel: [w542] -> w499 mode=indexing
                  tunnel: w503 -> [w545]
                  tunnel: w501 -> [w543]
                  tunnel: [w541] -> w500 mode=indexing
                  tunnel: [w541] -> w496
                  i -> [w546]
                  n237 = Divide(x=w546, y=w545) -> (x/y=w544:dbl)
                  n238 = Index Array(array=w547, index=w546) -> (element=w542:dbl)
                  n239 = Multiply(x=w544, y=w543) -> (x*y=w541:dbl)
                }
                n240 = case shown="True" w492 {
                  tunnel: w497 -> [_ w508]
                  tunnel: w496 -> [_ w509]
                  tunnel: w495 -> [_ w523]
                  tunnel: w494 -> [_ w511]
                  tunnel: w493 -> [_ w515]
                  frame False {
                  }
                  frame True {
                    n241 = Greater?(x=w508, y=w509) -> (0:w510:bool)
                    n242 = case shown="True" w510 {
                      tunnel: [w526 w527] -> w507
                      tunnel: w508 -> [w526 w533]
                      tunnel: w511 -> [_ w532]
                      tunnel: w509 -> [_ _]
                      tunnel: w508 -> [_ w531]
                      frame False {
                      }
                      frame True {
                        n243 = while {
                          tunnel: w532 -> [w540]
                          tunnel: w533 -> [w537]
                          shift-right: [w535] -> _
                          shift-left: w532 -> [w534]
                          shift-left: w532 -> [_]
                          tunnel: [w534] -> w530
                          i -> [w538]
                          stop <- w536 continue-if-true
                          n244 = Increment(x=w538) -> (x+1=w539:i32)
                          n245 = Multiply(x=w540, y=w539) -> (x*y=w535:dbl)
                          n246 = Greater?(x=w537, y=w535) -> (0:w536:bool)
                        }
                        n247 = Subtract(x=w530, y=w531) -> (x-y=w528:dbl)
                        n248 = Sign(1:w528) -> (0:w529:dbl)
                        n249 = Multiply(x=w528, y=w529) -> (x*y=w527:dbl)
                      }
                    }
                    n250 = Multiply(x=w523, y=w507) -> (x*y=w525:dbl)
                    n251 = local read "PSRR/CMRR Input"() -> (w521:T12)
                    n252 = Divide(x=w525, y=w511) -> (x/y=w524:dbl)
                    n253 = Unbundle By Name(w521) -> ("Bin Width"=w506:dbl)
                    n254 = To Long Integer(number=w524) -> (32bit integer=w520:i32)
                    n255 = Subtract(x=w520, y=w506) -> (x-y=w516:dbl)
                    n256 = Add(x=w520, y=w506) -> (x+y=w505:dbl)
                    n257 = Split 1D Array(array=w515, index=w505) -> (first subarray=w519:dbl[])  [unwired: 1 out]
                    n258 = Split 1D Array(array=w519, index=w516) -> (second subarray=w518:dbl[])  [unwired: 1 out]
                    n259 = Array Max & Min(array=w518) -> (max value=w514:dbl, max index (indices)=w517:i32)  [unwired: 2 out]
                    n260 = local read "PSRR/CMRR Output"() -> (w522:T11)
                    n261 = Add(x=w517, y=w516) -> (x+y=w513:dbl)
                    n262 = Bundle By Name(cluster=w522, "Ideal Power Bin"=w520, "Actual Power Bin"=w513, "Signal Strength (dB)"=w514) -> (→"PSRR/CMRR Output":T11)
                  }
                }
                n263 = Bundle(w500, w499) -> (→"FFT Plot":cluster{dbl[], dbl[]})  [unwired: 1 in]
              }
            }
          }
        }
        n264 = Build Array(w118, w119) -> (→"Raw_Histo":dbl[][])
      }
      frame "Cap Calib" {
        n265 = case shown="\"64\"" "Average Window" {
          tunnel: [8 16 32 64] -> w548
          frame "8", Default {
          }
          frame "16" {
          }
          frame "32" {
          }
          frame "64" {
          }
        }
        n266 = case shown="True" "Cap Calibration" {
          tunnel: w548 -> [_ w556]
          frame False {
          }
          frame True {
            n267 = local read "DNL Plot"() -> (w557:dbl[])
            n268 = local read "INL Plot"() -> (w558:dbl[])
            n269 = call "Cap_Calibration.vi"("INL"=w558, "DNL"=w557, "From File/ Waveform"="INL/DNL Values", "Select Channel"="Select Channel", "Average Window"=w556, "File path (DNL & INL)"="File path (DNL & INL)") -> ("ADC TEST 7"=→"ADC TEST 7":string, "ADC TEST 6"=→"ADC TEST 6":string, "ADC TEST 5"=→"ADC TEST 5":string, "Trim Coeff (Binary)"=→"Trim Coeff (Binary)":string[], "Trim Coeff (Integer)"=→"Trim Coeff (Integer)":dbl[])  [unwired: 1 in]
          }
        }
      }
      frame "Save data" {
        n270 = Unbundle By Name("path to save") -> ("Path to Save plot"=w568:path, "Path to Raw Data plot"=w571:path)
        n271 = disable-structure shown="Enabled" {
          disable-tunnel: w571 -> [w591 w709]
          disable-tunnel: [w583 w709] -> w569
          frame Disabled {
            w581 = "16Hits_Run" ("regular expression")
            n272 = local read "Run"() -> (w582:dbl)
            n273 = Increment(x=w582) -> (x+1=w586:dbl)
            n274 = local write "Run"(w586) -> ()
            n275 = Path To String(path=w591) -> (string=w590:string)
            n276 = Number To Decimal String(number=w586) -> (decimal integer string=w587:string)  [unwired: 1 in]
            n277 = xnode "Match Regular Expression"("input string"=w590, "regular expression"=w581) -> ("before match"=w589:string, "after match"=w588:string)  [unwired: 4 in, 3 out]
            n278 = Concatenate Strings(w581, w587) -> (w585:string)
            n279 = Concatenate Strings(w589, w585, w588) -> (w584:string)
            n280 = String To Path(string=w584) -> (path=w583:path)
          }
          frame Enabled {
          }
        }
        n281 = Unbundle By Name("Save data") -> ("Save INL/DNL Plot(Ramp)"=w577:bool, "Save INL/DNL Raw Data(Ramp)"=w576:bool, "Save INL/DNL Plot(Sine)"=w575:bool, "Save INL/DNL Raw Data(Sine)"=w574:bool, "Save SNR Plot"=w573:bool, "Save SNR Raw Data"=w572:bool, "Save DC Raw data"=w570:bool)  [unwired: 1 out]
        n282 = case shown="\"SNR\"" "Select the Tab to project" {
          tunnel: w568 -> [w713 w733 w757 _ _]
          tunnel: w569 -> [w714 w734 w756 _ w773]
          tunnel: w577 -> [w711 _ _ _ _]
          tunnel: w576 -> [w710 _ _ _ _]
          tunnel: w575 -> [_ w731 _ _ _]
          tunnel: w574 -> [_ w730 _ _ _]
          tunnel: w573 -> [_ _ w754 _ _]
          tunnel: w572 -> [_ _ w753 _ _]
          tunnel: w570 -> [_ _ _ _ w772]
          frame "ADC Ramp" {
            n283 = case shown="True" w711 {
              tunnel: w713 -> [_ w716]
              frame False {
              }
              frame True {
                n284 = Current VI's Path() -> (path=w717:path)
                n285 = call "Take fron panel screenshot.vi"("VI path"=w717, "Image path"=w716, "Visible area only? (f)"=FALSE, "File type (.jpg)"=enum16{".bmp", ".png", ".jpg"}.".png") -> ()  [unwired: 4 in, 1 out]
              }
            }
            n286 = case shown="True" w710 {
              tunnel: w714 -> [_ w723]
              frame False {
              }
              frame True {
                w722 = "" ("delimiter (\\t)")
                w721 = TRUE ("transpose? (no:F)")
                n287 = local read "Histogram waveform"() -> (w726:dbl[])
                n288 = local read "Ramp Waveform"() -> (w727:i64[])
                n289 = local read "DNL_Ramp"() -> (w729:dbl[])
                n290 = local read "INL_Ramp"() -> (w728:dbl[])
                n291 = call-poly <vilib>:"Write To Spreadsheet File.vi"("delimiter (\\t)"=w722, "1D data"=string[] ["ADC Raw data", "DNL", "INL", "Histogram"], "file path (dialog if empty)"=w723) -> ("new file path (Not A Path if cancelled)"=w724:path)  [unwired: 5 in]
                n292 = Build Array(w727, w729, w728, w726) -> (w725:dbl[][])
                n293 = call-poly <vilib>:"Write To Spreadsheet File.vi"("delimiter (\\t)"=w722, "transpose? (no:F)"=w721, "append to file? (new file:F)"=w721, "2D data"=w725, "file path (dialog if empty)"=w724) -> ()  [unwired: 3 in, 1 out]
              }
            }
            "Main Tab" <- 3 ("Select Tab")
            "Ramp" <- 2 ("Select Tab")
          }
          frame "ADC Sine", Default {
            n294 = case shown="True" w731 {
              tunnel: w733 -> [_ w736]
              frame False {
              }
              frame True {
                n295 = Current VI's Path() -> (path=w737:path)
                n296 = call "Take fron panel screenshot.vi"("VI path"=w737, "Image path"=w736, "Visible area only? (f)"=FALSE, "File type (.jpg)"=enum16{".bmp", ".png", ".jpg"}.".png") -> ()  [unwired: 4 in, 1 out]
              }
            }
